vi "TestRUSHClimb.vi"() -> ()   [LabVIEW 2012]
panel:
  out "Out Cluster":T1
  in  "ClimbDepEnable":bool
  in  "ClimbFoldEnable":bool
  in  "ClimbLimit":bool
  in  "ClimbExtEnable":bool
  in  "ClimbPOTDep":dbl(knob) scale=0.0..5.0
  in  "ClimbConst":T2={"ClimbConstDep"=0.7, "ClimbConstFold"=4.4, "ClimbConstExt"=4.0, "ClimbConstRet"=1.0}
  in  "ClimbPOTExt":dbl(slide) scale=0.0..5.0
  in  "ClimbRetEnable":bool
  in  "ClimbManualDep":dbl(slide) scale=-1.0..1.0
  in  "ClimbManualExt":dbl(slide) scale=-1.0..1.0
  in  "In Cluster":T3
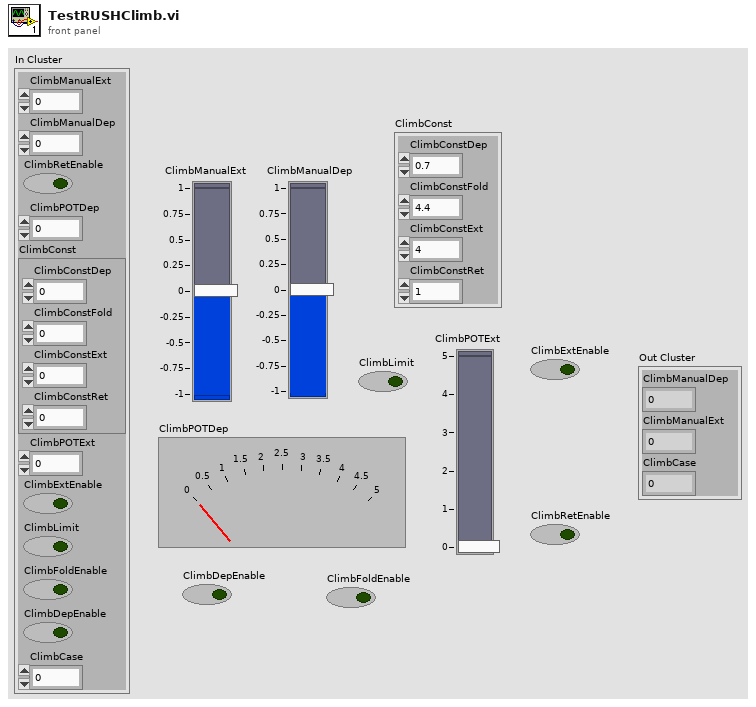
[diagram p1: front panel]
types:
  T1 = cluster{"ClimbManualDep":dbl, "ClimbManualExt":dbl, "ClimbCase":i32}
  T2 = cluster{"ClimbConstDep":dbl, "ClimbConstFold":dbl, "ClimbConstExt":dbl, "ClimbConstRet":dbl}
  T3 = cluster{"ClimbManualExt":dbl, "ClimbManualDep":dbl, "ClimbRetEnable":bool, "ClimbPOTDep":dbl, "ClimbConst":cluster{"ClimbConstDep":dbl, "ClimbConstFold":dbl, "ClimbConstExt":dbl, "ClimbConstRet":dbl}, "ClimbPOTExt":dbl, "ClimbExtEnable":bool, "ClimbLimit":bool, "ClimbFoldEnable":bool, "ClimbDepEnable":bool, "ClimbCase":dbl}
  T4 = cluster{"ClimbOutDep":dbl, "ClimbOutExt":dbl, "ClimbOutCase":i32}
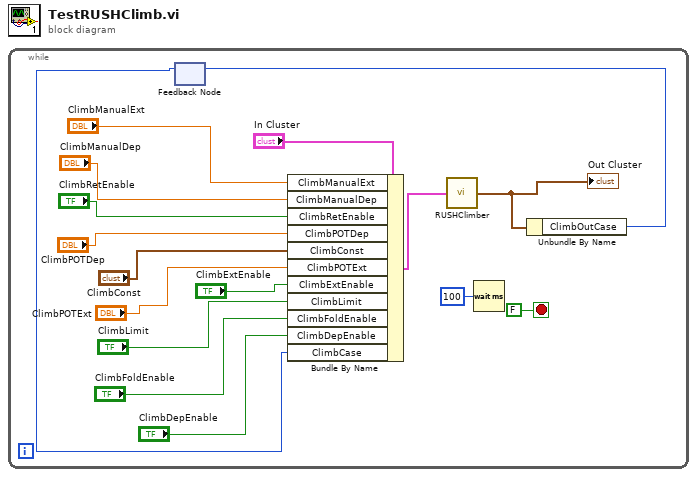
[diagram p0: block diagram]
diagram:
  n1 = while {
    stop <- FALSE stop-if-true
    n2 = feedback #1() -> (w3:i32)  [unwired: 1 in]
    n3 = Bundle By Name(cluster="In Cluster", "ClimbManualExt"="ClimbManualExt", "ClimbManualDep"="ClimbManualDep", "ClimbRetEnable"="ClimbRetEnable", "ClimbPOTDep"="ClimbPOTDep", "ClimbConst"="ClimbConst", "ClimbPOTExt"="ClimbPOTExt", "ClimbExtEnable"="ClimbExtEnable", "ClimbLimit"="ClimbLimit", "ClimbFoldEnable"="ClimbFoldEnable", "ClimbDepEnable"="ClimbDepEnable", "ClimbCase"=w3) -> (w15:T3)
    n4 = call "RUSHClimber.vi"("In Cluster"=w15) -> ("Out Cluster"=w6:T4)
    "Out Cluster" <- w6
    n5 = Wait (ms)(milliseconds to wait=u32 100) -> ()  [unwired: 1 out]
    n6 = Unbundle By Name(w6) -> ("ClimbOutCase"=w4:i32)
    n7 = feedback-in #1(w4) -> ()
  }
